vi "Display.vi"(8 "error in":errorcluster, 11 "Timeout Two Button in":refnum<class "SVG - Timeout Two Button.lvclass">) -> (0 "error out":errorcluster, 3 "Timeout Two Button out":refnum<class "SVG - Timeout Two Button.lvclass">)   [LabVIEW 2021, in "Pop-Up.lvlib" / "SVG - Timeout Two Button.lvclass"]
doc: "This vi displays the custom image two button timeout popup.\n\n<b>Code Developed By:</b>\nDaniel Coons\nTechnology Service Corporation\n1983 S Liberty Drive\nBloomington, IN 47403\nPhone: 812 558-7100\ndaniel.coons@tsc.com\nwww.tsc.com"
uses:
  SVG - Timeout Two Button.lvclass
  C:/Development/TSC.Pop-Up/Popup/Popup.lvclass
  <vilib>/Utility/miscctls.llb/LVPositionTypeDef.ctl
  SVG - Timeout Two Button.lvclass/SVG - Timeout Two Button.ctl
  Popup/Popup.lvclass/Popup.ctl
  Popup/Data Member Access/Read Theme.vi
  Theme/Theme.lvclass
  Popup/Popup.lvclass
  C:/Development/TSC.Pop-Up/SVG/SVG Parent.lvclass
  C:/Development/TSC.Pop-Up/SVG/Custom/SVG - Timeout Two Button/SVG - Timeout Two Button.lvclass
  user32.dll
panel:
  out "header":bool
  out "count":string
  in  "n-text":bool
  in  "y-text":bool
  out "2D Picture":picture
  out "Message":string
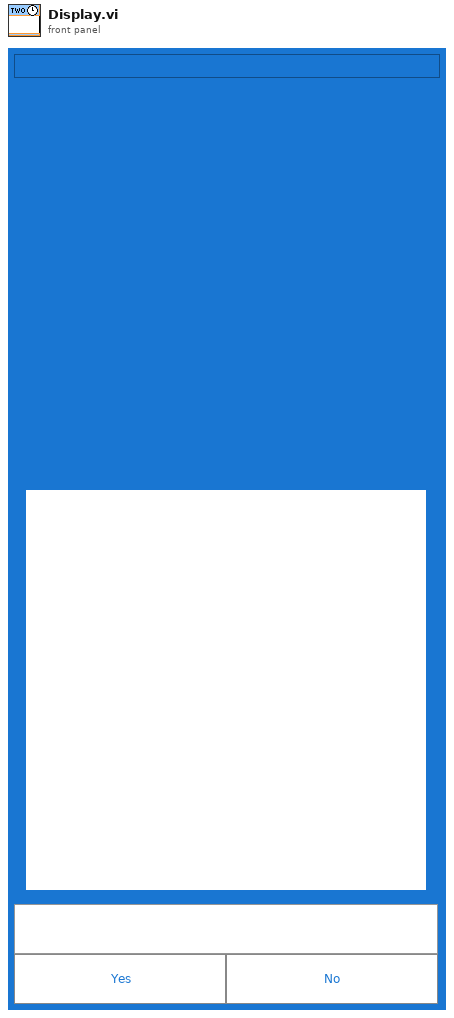
[diagram p1: front panel]
types:
  T1 = typedef "LVPositionTypeDef.ctl" = cluster{"Left":i32, "Top":i32}
  T2 = typedef "LVPoint32TypeDef.ctl" = cluster{"Horizontal":i32, "Vertical":i32}
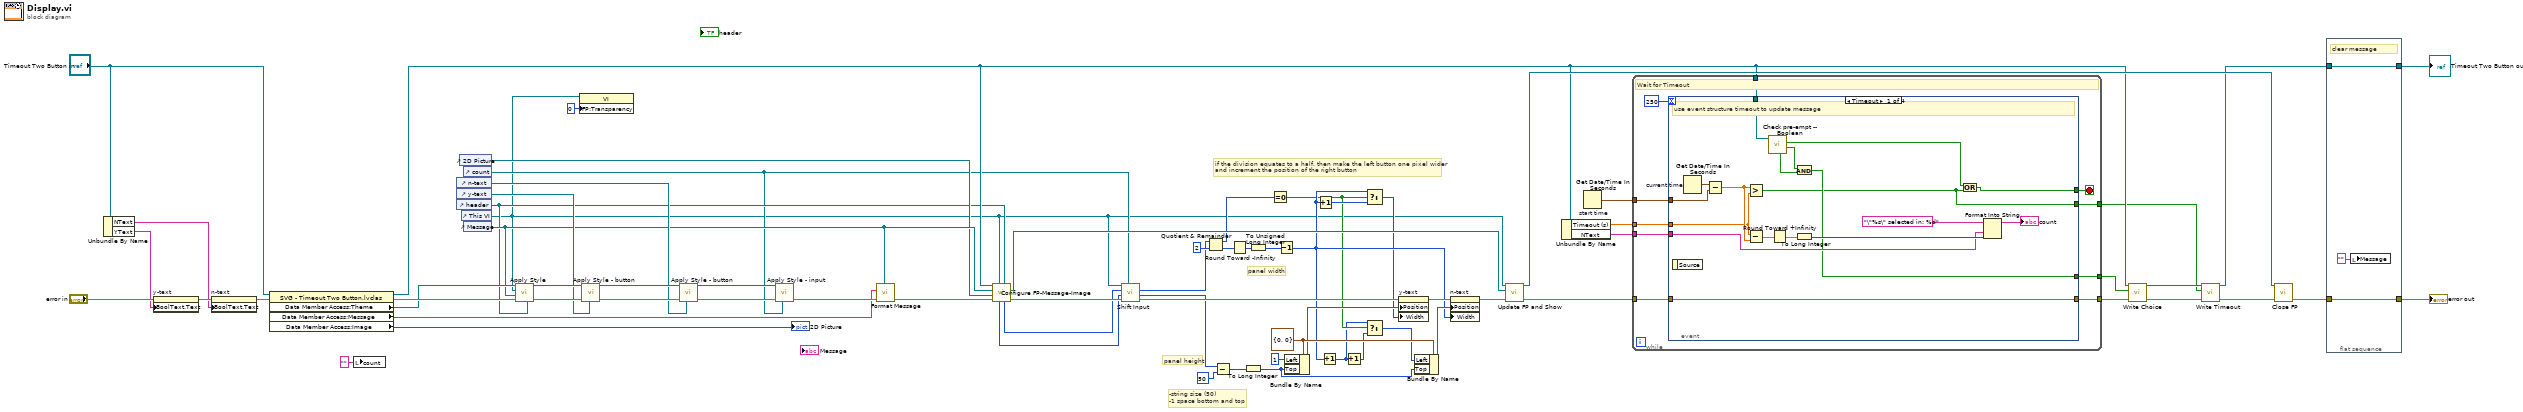
[diagram p0: block diagram]
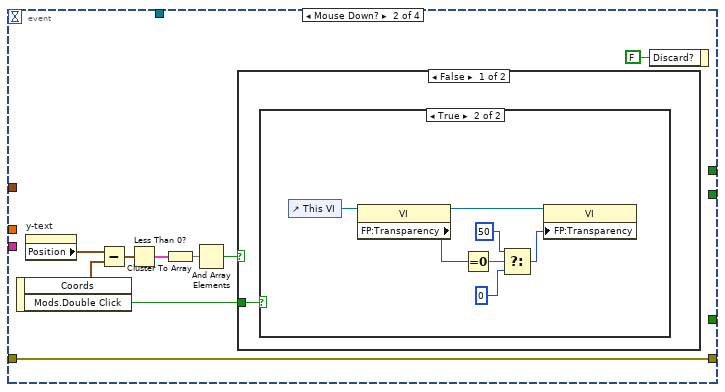
[diagram p2: hidden frame]
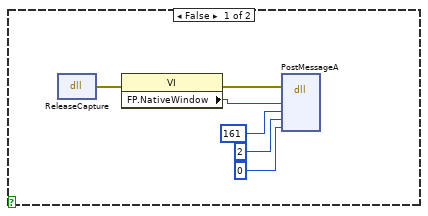
[diagram p3: hidden frame]
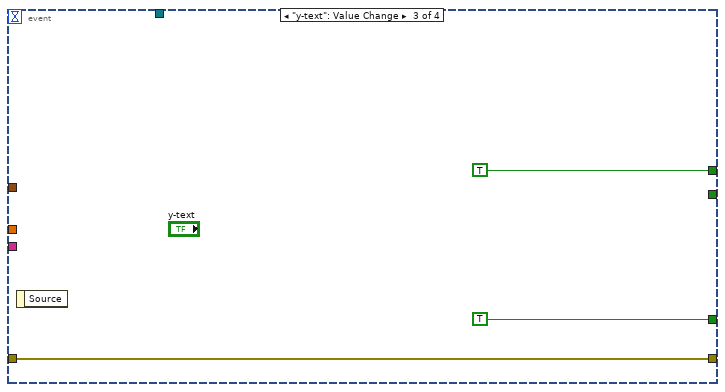
[diagram p5: hidden frame]
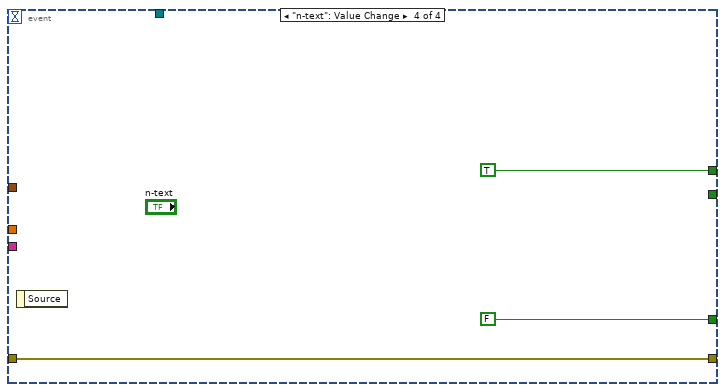
[diagram p6: hidden frame]
diagram:
  w40 = T1 {"Left"=0, "Top"=0} ("Position")
  # "if the division equates to a half, then make the left button one pixel wider \nand increment the position of the right button"
  # "-string size (50)\n-1 space bottom and top"
  # "panel width"
  # "panel height"
  n1 = Unbundle By Name("Timeout Two Button in") -> ("NText"=w66:string, "YText"=w68:string)
  n2 = property on="y-text" class="Bool"(error in="error in", "BoolText.Text"=w68) -> (error out=w69:errorcluster)  [unwired: 1 in, 1 out]
  n3 = property on="n-text" class="Bool"(error in=w69, "BoolText.Text"=w66) -> (error out=w67:errorcluster)  [unwired: 1 in, 1 out]
  n4 = property class="SVG - Timeout Two Button.lvclas"(reference="Timeout Two Button in", error in=w67) -> (reference out=w25:refnum<class "SVG - Timeout Two Button.lvclass">, error out=w53:errorcluster, "Data Member Access:Theme"=w51:refnum<class "Theme.lvclass">, "Data Member Access:Message"=w42:string, "Data Member Access:Image"=→"2D Picture":picture)
  n5 = local write "count"("" ("count")) -> ()
  n6 = control-ref of="n-text"() -> (w45:refnum<vi>)
  n7 = control-ref of="y-text"() -> (w46:refnum<vi>)
  n8 = control-ref of="header"() -> (w22:refnum<vi>)
  n9 = control-ref of="2D Picture"() -> (w23:refnum<vi>)
  n10 = control-ref of="This VI"() -> (w6:refnum<vi>)
  n11 = control-ref of="count"() -> (w19:refnum<vi>)
  n12 = control-ref of="Message"() -> (w24:refnum<vi>)
  n13 = call "Apply Style.vi"("header ref"=w22, "error in (no error)"=w53, "message ref"=w24, "pop up ref"=w6, "Theme in"=w51) -> ("error out"=w52:errorcluster, "Theme out"=w47:refnum<class "Theme.lvclass">)  [unwired: 5 in]
  n14 = property class="VI"(reference=w6, "FP:Transparency"=u8 0 ("Front Panel Window:Transparency")) -> ()  [unwired: 1 in, 2 out]
  n15 = call "Apply Style - button.vi"("button ref"=w46, "error in (no error)"=w52, "Theme in"=w47) -> ("error out"=w50:errorcluster, "Theme out"=w48:refnum<class "Theme.lvclass">)  [unwired: 7 in]
  n16 = call "Apply Style - button.vi"("button ref"=w45, "error in (no error)"=w50, "Theme in"=w48) -> ("error out"=w49:errorcluster, "Theme out"=w43:refnum<class "Theme.lvclass">)  [unwired: 7 in]
  n17 = call "Apply Style - input.vi"("input ref"=w19, "error in (no error)"=w49, "Theme in"=w43) -> ("error out"=w44:errorcluster)  [unwired: 7 in, 1 out]
  n18 = call "Format Message.vi"("formatted string"=w24, "error in"=w44, "String Input"=w42) -> ("error out"=w27:errorcluster)  [unwired: 7 in, 1 out]
  n19 = call "Configure FP-Message-Image.vi"("header ref"=w22, "Pop Up ref"=w6, "error in (no error)"=w27, "Image ref"=w23, "Message ref"=w24, "Popup in"=w25) -> ("error out"=w28:errorcluster, "Panel Ref"=w21:refnum<vi>, "Panel Width"=w18:i32, "Panel Height"=w16:i32)  [unwired: 1 in, 1 out]
  n20 = call "Shift Input.vi"("Control"=w19, "Error In"=w28, "Panel Height"=w16, "Panel Width"=w18, "Pop Up ref"=w6) -> ("Error Out"=w20:errorcluster, "Panel Height out"=w15:i32, "Panel Width out"=w17:i32)  [unwired: 4 in]
  n21 = Quotient & Remainder(x=w17, y=2) -> (x-y*floor(x/y)=w14:i32, floor(x/y)=w32:i32)
  n22 = Subtract(x=w15, y=50 ("value")) -> (x-y=w35:i32)
  n23 = Round Toward -Infinity(1:w32) -> (0:w29:i32)
  n24 = To Long Integer(number=w35) -> (32bit integer=w38:i32)
  n25 = To Unsigned Long Integer(number=w29) -> (unsigned 32bit integer=w30:u32)
  n26 = Equal To 0?(x=w14) -> (x = 0?=w10:bool)
  n27 = Decrement(x=w30) -> (x-1=w13:u32)
  n28 = Bundle By Name(cluster=w40, "Left"=1, "Top"=w38) -> (w36:T1)
  n29 = Increment(x=w13) -> (x+1=w12:u32)
  n30 = Increment(x=w13) -> (x+1=w9:u32)
  n31 = Increment(x=w9) -> (x+1=w8:u32)
  n32 = Select(t=w13, s=w10, f=w12) -> (s? t:f=w11:u32)
  n33 = Select(t=w9, s=w10, f=w8) -> (s? t:f=w7:u32)
  n34 = property on="y-text" class="Bool"(error in=w20, "Position"=w36, "Width"=w11) -> (error out=w37:errorcluster)  [unwired: 1 in, 1 out]
  n35 = Bundle By Name(cluster=w40, "Left"=w7, "Top"=w38) -> (w39:T1)
  n36 = property on="n-text" class="Bool"(error in=w37, "Position"=w39, "Width"=w13) -> (error out=w26:errorcluster)  [unwired: 1 in, 1 out]
  n37 = call "Update FP and Show.vi"("error in (no error)"=w26, "Panel Ref"=w21, "VI in"=w6) -> ("error out"=w65:errorcluster, "VI out"=w55:refnum<vi>)  [unwired: 7 in]
  n38 = Unbundle By Name(w25) -> ("Timeout (s)"=w63:dbl, "NText"=w62:string)
  n39 = Get Date/Time In Seconds "start time"() -> (seconds since 1Jan1904=w64:timestamp)
  n40 = while {
    tunnel: [w76] -> w61
    tunnel: w65 -> [w77]
    tunnel: w64 -> [w81]
    tunnel: w63 -> [w79]
    tunnel: w62 -> [w75]
    tunnel: [w74] -> w60
    tunnel: w25 -> [w73]
    tunnel: [w72] -> w1
    stop <- w80 stop-if-true
    # "Wait for Timeout"
    n41 = event shown="[0] Timeout" {
      selector: _ -> [_ _ _ _]
      dyn-events: _ -> [_ _ _ _]
      timeout: 250 -> [_ _ _ _]
      tunnel: w81 -> [w99 _ _ _]
      tunnel: [w89 _ TRUE TRUE] -> w80
      tunnel: w79 -> [w95 _ _ _]
      tunnel: w77 -> [w93 w107 w125 w128]
      tunnel: [w93 w107 w125 w128] -> w76
      tunnel: w75 -> [w91 _ _ _]
      tunnel: [w85 _ TRUE FALSE] -> w74
      tunnel: w73 -> [w90 _ _ _]
      tunnel: [w82 _ _ _] -> w72
      event Timeout {
        # "use event structure timeout to update message"
        n42 = event-data() -> ()  [unwired: 1 in, 1 out]
        n43 = Get Date/Time In Seconds "current time"() -> (seconds since 1Jan1904=w98:timestamp)
        n44 = Subtract(x=w98, y=w99) -> (x-y=w97:dbl)
        n45 = Greater?(x=w97, y=w95) -> (0:w82:bool)
        n46 = Subtract(x=w95, y=w97) -> (x-y=w96:dbl)
        n47 = call "Check pre-empt -- Boolean.vi"("_Popup in"=w90) -> ("Value?"=w87:bool, "Pre-empted?"=w88:bool, "Type Match?"=w86:bool)  [unwired: 7 in, 1 out]
        n48 = Round Toward +Infinity(x=w96) -> (ceil(x): smallest int >= x=w83:dbl)
        n49 = And(x=w87, y=w86) -> (x .and. y?=w85:bool)
        n50 = To Long Integer(number=w83) -> (32bit integer=w92:i32)
        n51 = Or(x=w88, y=w82) -> (x .or. y?=w89:bool)
        n52 = Format Into String(format string="\"%s\" selected in: %d", w91, w92) -> (resulting string=→"count":string)  [unwired: 2 in, 1 out]
      }
      event Mouse Down? {
        n53 = event-data() -> ("Coords"=w100:T2, "Mods.Double Click"=w101:bool)  [unwired: 1 in]
        n54 = property on="y-text" class="Bool"() -> ("Position"=w106:T1)  [unwired: 2 in, 2 out]
        n55 = Subtract(x=w106, y=w100) -> (x-y=w105:T1)
        n56 = Less Than 0?(x=w105) -> (x < 0?=w104:cluster{"Left":bool, "Top":bool})
        n57 = Cluster To Array(cluster=w104) -> (array=w103:bool[])
        n58 = And Array Elements(Boolean array=w103) -> (logical AND=w102:bool)
        n59 = case shown="False" w102 {
          tunnel: w101 -> [w109 _]
          frame False {
            n60 = case shown="True" w109 {
              frame False {
                n61 = dll-call lib="user32.dll" fn="ReleaseCapture"() -> (error out=w113:errorcluster)  [unwired: 4 in, 1 out]
                n62 = property class="VI"(error in=w113) -> (error out=w114:errorcluster, "FP.NativeWindow"=w115:u64)  [unwired: 1 in, 1 out]
                n63 = dll-call lib="user32.dll" fn="PostMessageA"(error in=w114, "hWnd"=w115, "Msg"=161, "wParam"=2, "lParam"=0) -> ()  [unwired: 7 in, 2 out]
              }
              frame True {
                n64 = control-ref of="This VI"() -> (w122:refnum<vi>)
                n65 = property class="VI"(reference=w122) -> (reference out=w120:refnum<vi>, "FP:Transparency"=w121:u8)  [unwired: 1 in, 1 out]
                n66 = Equal To 0?(x=w121) -> (x = 0?=w119:bool)
                n67 = Select(t=u8 50, s=w119, f=u8 0) -> (s? t:f=w118:u8)
                n68 = property class="VI"(reference=w120, "FP:Transparency"=w118) -> ()  [unwired: 1 in, 2 out]
              }
            }
          }
          frame True {
          }
        }
        n69 = event-data("Discard?"=FALSE) -> ()  [unwired: 1 in, 1 out]
      }
      event "y-text": Value Change {
        n70 = event-data() -> ()  [unwired: 1 in, 1 out]
      }
      event "n-text": Value Change {
        n71 = event-data() -> ()  [unwired: 1 in, 1 out]
      }
    }
  }
  n72 = call-dynamic "Write Choice.vi"("error in (no error)"=w61, "Choice"=w60, "_Popup in"=w25) -> ("error out"=w58:errorcluster, "_Popup out"=w3:refnum<class "SVG - Timeout Two Button.lvclass">)  [unwired: 7 in]
  n73 = call "Write Timeout.vi"("error in (no error)"=w58, "Timeout?"=w1, "Popup in"=w3) -> ("error out"=w4:errorcluster, "Popup out"=w2:refnum<class "SVG - Timeout Two Button.lvclass">)  [unwired: 7 in]
  n74 = call "Close FP.vi"("error in (no error)"=w4, "VI in"=w55) -> ("error out"=w59:errorcluster)  [unwired: 9 in]
  n75 = flat-sequence {
    tunnel: w59 -> [w131]
    tunnel: [w131] -> w57
    tunnel: w2 -> [w130]
    tunnel: [w130] -> w56
    frame #0 {
      # "clear message"
      n76 = local write "Message"("" ("Message")) -> ()
    }
  }
  "error out" <- w57
  "Timeout Two Button out" <- w56
